vi "get_TIFF_number_of_pages.vi"(8 "error in (no error)":errorcluster, 11 "path in":path) -> (0 "error out":errorcluster, 2 "number of pages":i32, 3 "path out":path)   [LabVIEW 2010, in "TIFFManagement.lvlib"]
uses:
  TIFFManagement.lvlib
  VisualCPP/Release/TIFFManagement.dll
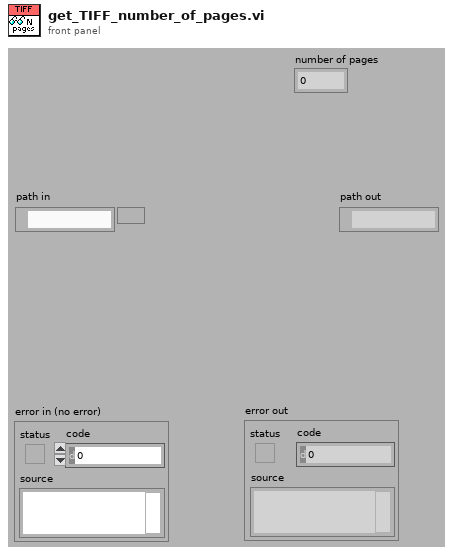
[diagram p1: front panel]
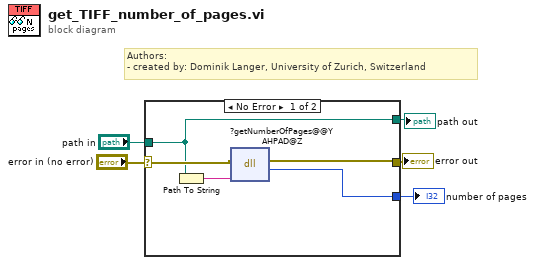
[diagram p0: block diagram]
diagram:
  # "Authors: \n- created by: Dominik Langer, University of Zurich, Switzerland"
  n1 = case shown="No Error" "error in (no error)" {
    selector: "error in (no error)" -> [w9 w12]
    tunnel: "path in" -> [w6 w11]
    tunnel: [w8 w12] -> w3
    tunnel: [w6 w11] -> w2
    tunnel: [w7 _] -> w1
    frame No Error {
      n2 = Path To String(path=w6) -> (string=w10:string)
      n3 = dll-call lib="C:/helioscan/common/libraries/TIFFManagement/VisualCPP/Release/TIFFManagement.dll" fn="?getNumberOfPages@@YAHPAD@Z"(error in=w9, "path"=w10) -> (error out=w8:errorcluster, "return type"=w7:i32)  [unwired: 3 in, 1 out]
    }
    frame Error {
    }
  }
  "error out" <- w3
  "path out" <- w2
  "number of pages" <- w1
